vi "Spartan HTTP Write Reply.vi"(8 "error in (no error)":errorcluster, 9 "content":string, 10 "header":string, 11 "http session":T1 {"object data"."time" format="%0.2f"}) -> (0 "error out":errorcluster)   [LabVIEW 2011]
doc: "Writes a reply to the HTTP connections that the <B>cgi connection info</B> input specifies."
uses:
  Spartan HTTP Session.ctl
  ITK EXT/http/http_obj.llb/HTTP Session Data.ctl
  ITK EXT/utils/keyedarr.llb/Keyed Array.ctl
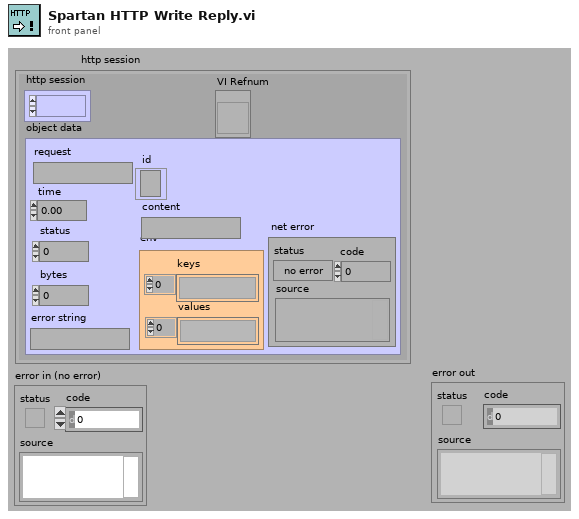
[diagram p1: front panel]
types:
  T1 = typedef "Spartan HTTP Session.ctl" = cluster{"http session":refnum<k1>, "object data":T2, "VI Refnum":refnum<vi>}
  T2 = typedef "HTTP Session Data.ctl" = cluster{"request":string, "time":dbl, "status":i32, "error string":string, "bytes":i32, "env":T3, "content":string, "id":refnum<k5>, "net error":errorcluster}
  T3 = typedef "Keyed Array.ctl" = cluster{"keys":string[], "values":string[]}
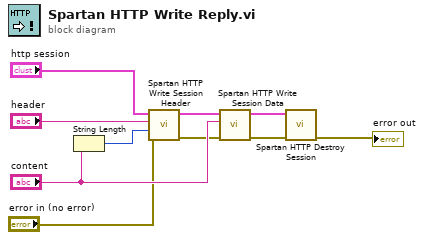
[diagram p0: block diagram]
diagram:
  n1 = String Length(string="content") -> (length=w5:i32)
  n2 = call "Spartan HTTP Write Session Header.vi"("error in (no error)"="error in (no error)", "content length (-1)"=w5, "header"="header", "http session"="http session") -> ("error out"=w6:errorcluster, "http session out"=w8:T1)  [unwired: 1 in, 5 out]
  n3 = call "Spartan HTTP Write Session Data.vi"("error in (no error)"=w6, "data"="content", "http session"=w8) -> ("error out"=w2:errorcluster, "http session out"=w3:T1)  [unwired: 3 out]
  n4 = call "Spartan HTTP Destroy Session.vi"("error in (no error)"=w2, "object"=w3) -> ("error out"=→"error out":errorcluster)  [unwired: 1 in, 8 out]
